vi "WriteTables1212(Host).vi"(1 "Select Channel":u16(ring) items=["CH 1", "CH 2"], 2 "WavefArray":u16[](array[numeric])=[8192, 8210, 8229, 8247, 8266, 8284, 8302, 8321, 8339, 8358, 8376, 8394, 8413, 8431, 8450, 8468, 8486, 8505, 8523, 8542, 8560, 8578, 8597, 8615, 8633, 8652, 8670, 8688, 8707, 8725, 8743, 8762, 8780, 8798, 8817, 8835, 8853, 8872, 8890, 8908, 8926, 8945, 8963, 8981, 8999, 9018, 9036, 9054, 9072, 9091, 9109, 9127, 9145, 9163, 9181, 9200, 9218, 9236, 9254, 9272, 9290, 9308, 9326, 9344, 9363, 9381, 9399, 9417, 9435, 9453, 9471, 9489, 9507, 9525, 9543, 9560, 9578, 9596, 9614, 9632, 9650, 9668, 9686, 9703, 9721, 9739, 9757, 9775, 9792, 9810, 9828, 9845, 9863, 9881, 9898, 9916, 9934, 9951, 9969, 9986, 10004, 10022, 10039, 10057, 10074, 10092, 10109, 10126, 10144, 10161, 10179, 10196, 10213, 10231, 10248, 10265, 10283, 10300, 10317, 10334, 10351, 10369, 10386, 10403, 10420, 10437, 10454, 10471, 10488, 10505, 10522, 10539, 10556, 10573, 10590, 10607, 10623, 10640, 10657, 10674, 10691, 10707, 10724, 10741, 10757, 10774, 10791, 10807, 10824, 10840, 10857, 10873, 10890, 10906, 10923, 10939, 10955, 10972, 10988, 11004, 11020, 11037, 11053, 11069, 11085, 11101, 11117, 11133, 11149, 11165, 11181, 11197, 11213, 11229, 11245, 11261, 11277, 11292, 11308, 11324, 11340, 11355, 11371, 11386, 11402, 11418, 11433, 11449, 11464, 11479, 11495, 11510, 11525, 11541, 11556, 11571, 11586, 11602, 11617, 11632, 11647, 11662, 11677, 11692, 11707, 11722, 11737, 11751, 11766, 11781, 11796, 11810, 11825, 11840, 11854, 11869, 11883, 11898, 11912, 11927, 11941, 11956, 11970, 11984, 11998, 12013, 12027, 12041, 12055, 12069, 12083, 12097, 12111, 12125, 12139, 12153, 12166, 12180, 12194, 12208, 12221, 12235, 12249, 12262, 12276, 12289, 12303, 12316, 12329, 12343, 12356, 12369, 12382, 12395, 12409, 12422, 12435, 12448, 12461, 12474, 12486, 12499, 12512, 12525, 12537, 12550, 12563, 12575, 12588, 12600, 12613, 12625, 12638, 12650, 12662, 12675, 12687, 12699, 12711, 12723, 12735, 12747, 12759, 12771, 12783, 12795, 12807, 12818, 12830, 12842, 12853, 12865, 12876, 12888, 12899, 12911, 12922, 12933, 12945, 12956, 12967, 12978, 12989, 13000, 13011, 13022, 13033, 13044, 13055, 13066, 13076, 13087, 13098, 13108, 13119, 13129, 13140, 13150, 13160, 13171, 13181, 13191, 13201, 13211, 13221, 13231, 13241, 13251, 13261, 13271, 13281, 13290, 13300, 13310, 13319, 13329, 13338, 13348, 13357, 13367, 13376, 13385, 13394, 13403, 13413, 13422, 13431, 13440, 13448, 13457, 13466, 13475, 13484, 13492, 13501, 13509, 13518, 13526, 13535, 13543, 13551, 13560, 13568, 13576, 13584, 13592, 13600, 13608, 13616, 13624, 13632, 13639, 13647, 13655, 13662, 13670, 13677, 13685, 13692, 13699, 13707, 13714, 13721, 13728, 13735, 13742, 13749, 13756, 13763, 13770, 13777, 13783, 13790, 13797, 13803, 13810, 13816, 13822, 13829, 13835, 13841, 13847, 13854, 13860, 13866, 13872, 13878, 13883, 13889, 13895, 13901, 13906, 13912, 13917, 13923, 13928, 13934, 13939, 13944, 13949, 13955, 13960, 13965, 13970, 13975, 13980, 13984, 13989, 13994, 13999, 14003, 14008, 14012, 14017, 14021, 14025, 14030, 14034, 14038, 14042, 14046, 14050, 14054, 14058, 14062, 14066, 14069, 14073, 14077, 14080, 14084, 14087, 14091, 14094, 14097, 14100, 14104, 14107, 14110, 14113, 14116, 14119, 14122, 14124, 14127, 14130, 14132, 14135, 14137, 14140, 14142, 14145, 14147, 14149, 14151, 14153, 14155, 14157, 14159, 14161, 14163, 14165, 14167, 14168, 14170, 14171, 14173, 14174, 14176, 14177, 14178, 14180, 14181, 14182, 14183, 14184, 14185, 14186, 14186, 14187, 14188, 14189, 14189, 14190, 14190, 14191, 14191, 14191, 14192, 14192, 14192, 14192, 14192, 14192, 14192, 14192, 14192, 14191, 14191, 14191, 14190, 14190, 14189, 14189, 14188, 14187, 14186, 14186, 14185, 14184, 14183, 14182, 14181, 14180, 14178, 14177, 14176, 14174, 14173, 14171, 14170, 14168, 14167, 14165, 14163, 14161, 14159, 14157, 14155, 14153, 14151, 14149, 14147, 14145, 14142, 14140, 14137, 14135, 14132, 14130, 14127, 14124, 14122, 14119, 14116, 14113, 14110, 14107, 14104, 14100, 14097, 14094, 14091, 14087, 14084, 14080, 14077, 14073, 14069, 14066, 14062, 14058, 14054, 14050, 14046, 14042, 14038, 14034, 14030, 14025, 14021, 14017, 14012, 14008, 14003, 13999, 13994, 13989, 13984, 13980, 13975, 13970, 13965, 13960, 13955, 13949, 13944, 13939, 13934, 13928, 13923, 13917, 13912, 13906, 13901, 13895, 13889, 13883, 13878, 13872, 13866, 13860, 13854, 13847, 13841, 13835, 13829, 13822, 13816, 13810, 13803, 13797, 13790, 13783, 13777, 13770, 13763, 13756, 13749, 13742, 13735, 13728, 13721, 13714, 13707, 13699, 13692, 13685, 13677, 13670, 13662, 13655, 13647, 13639, 13632, 13624, 13616, 13608, 13600, 13592, 13584, 13576, 13568, 13560, 13551, 13543, 13535, 13526, 13518, 13509, 13501, 13492, 13484, 13475, 13466, 13457, 13448, 13440, 13431, 13422, 13413, 13403, 13394, 13385, 13376, 13367, 13357, 13348, 13338, 13329, 13319, 13310, 13300, 13290, 13281, 13271, 13261, 13251, 13241, 13231, 13221, 13211, 13201, 13191, 13181, 13171, 13160, 13150, 13140, 13129, 13119, 13108, 13098, 13087, 13076, 13066, 13055, 13044, 13033, 13022, 13011, 13000, 12989, 12978, 12967, 12956, 12945, 12933, 12922, 12911, 12899, 12888, 12876, 12865, 12853, 12842, 12830, 12818, 12807, 12795, 12783, 12771, 12759, 12747, 12735, 12723, 12711, 12699, 12687, 12675, 12662, 12650, 12638, 12625, 12613, 12600, 12588, 12575, 12563, 12550, 12537, 12525, 12512, 12499, 12486, 12474, 12461, 12448, 12435, 12422, 12409, 12395, 12382, 12369, 12356, 12343, 12329, 12316, 12303, 12289, 12276, 12262, 12249, 12235, 12221, 12208, 12194, 12180, 12166, 12153, 12139, 12125, 12111, 12097, 12083, 12069, 12055, 12041, 12027, 12013, 11998, 11984, 11970, 11956, 11941, 11927, 11912, 11898, 11883, 11869, 11854, 11840, 11825, 11810, 11796, 11781, 11766, 11751, 11737, 11722, 11707, 11692, 11677, 11662, 11647, 11632, 11617, 11602, 11586, 11571, 11556, 11541, 11525, 11510, 11495, 11479, 11464, 11449, 11433, 11418, 11402, 11386, 11371, 11355, 11340, 11324, 11308, 11292, 11277, 11261, 11245, 11229, 11213, 11197, 11181, 11165, 11149, 11133, 11117, 11101, 11085, 11069, 11053, 11037, 11020, 11004, 10988, 10972, 10955, 10939, 10923, 10906, 10890, 10873, 10857, 10840, 10824, 10807, 10791, 10774, 10757, 10741, 10724, 10707, 10691, 10674, 10657, 10640, 10623, 10607, 10590, 10573, 10556, 10539, 10522, 10505, 10488, 10471, 10454, 10437, 10420, 10403, 10386, 10369, 10351, 10334, 10317, 10300, 10283, 10265, 10248, 10231, 10213, 10196, 10179, 10161, 10144, 10126, 10109, 10092, 10074, 10057, 10039, 10022, 10004, 9986, 9969, 9951, 9934, 9916, 9898, 9881, 9863, 9845, 9828, 9810, 9792, 9775, 9757, 9739, 9721, 9703, 9686, 9668, 9650, 9632, 9614, 9596, 9578, 9560, 9543, 9525, 9507, 9489, 9471, 9453, 9435, 9417, 9399, 9381, 9363, 9344, 9326, 9308, 9290, 9272, 9254, 9236, 9218, 9200, 9181, 9163, 9145, 9127, 9109, 9091, 9072, 9054, 9036, 9018, 8999, 8981, 8963, 8945, 8926, 8908, 8890, 8872, 8853, 8835, 8817, 8798, 8780, 8762, 8743, 8725, 8707, 8688, 8670, 8652, 8633, 8615, 8597, 8578, 8560, 8542, 8523, 8505, 8486, 8468, 8450, 8431, 8413, 8394, 8376, 8358, 8339, 8321, 8302, 8284, 8266, 8247, 8229, 8210, 8192, 8174, 8155, 8137, 8118, 8100, 8082, 8063, 8045, 8026, 8008, 7990, 7971, 7953, 7934, 7916, 7898, 7879, 7861, 7842, 7824, 7806, 7787, 7769, 7751, 7732, 7714, 7696, 7677, 7659, 7641, 7622, 7604, 7586, 7567, 7549, 7531, 7512, 7494, 7476, 7458, 7439, 7421, 7403, 7385, 7366, 7348, 7330, 7312, 7293, 7275, 7257, 7239, 7221, 7203, 7184, 7166, 7148, 7130, 7112, 7094, 7076, 7058, 7040, 7021, 7003, 6985, 6967, 6949, 6931, 6913, 6895, 6877, 6859, 6841, 6824, 6806, 6788, 6770, 6752, 6734, 6716, 6698, 6681, 6663, 6645, 6627, 6609, 6592, 6574, 6556, 6539, 6521, 6503, 6486, 6468, 6450, 6433, 6415, 6398, 6380, 6362, 6345, 6327, 6310, 6292, 6275, 6258, 6240, 6223, 6205, 6188, 6171, 6153, 6136, 6119, 6101, 6084, 6067, 6050, 6033, 6015, 5998, 5981, 5964, 5947, 5930, 5913, 5896, 5879, 5862, 5845, 5828, 5811, 5794, 5777, 5761, 5744, 5727, 5710, 5693, 5677, 5660, 5643, 5627, 5610, 5593, 5577, 5560, 5544, 5527, 5511, 5494, 5478, 5461, 5445, 5429, 5412, 5396, 5380, 5364, 5347, 5331, 5315, 5299, 5283, 5267, 5251, 5235, 5219, 5203, 5187, 5171, 5155, 5139, 5123, 5107, 5092, 5076, 5060, 5044, 5029, 5013, 4998, 4982, 4966, 4951, 4935, 4920, 4905, 4889, 4874, 4859, 4843, 4828, 4813, 4798, 4782, 4767, 4752, 4737, 4722, 4707, 4692, 4677, 4662, 4647, 4633, 4618, 4603, 4588, 4574, 4559, 4544, 4530, 4515, 4501, 4486, 4472, 4457, 4443, 4428, 4414, 4400, 4386, 4371, 4357, 4343, 4329, 4315, 4301, 4287, 4273, 4259, 4245, 4231, 4218, 4204, 4190, 4176, 4163, 4149, 4135, 4122, 4108, 4095, 4081, 4068, 4055, 4041, 4028, 4015, 4002, 3989, 3975, 3962, 3949, 3936, 3923, 3910, 3898, 3885, 3872, 3859, 3847, 3834, 3821, 3809, 3796, 3784, 3771, 3759, 3746, 3734, 3722, 3709, 3697, 3685, 3673, 3661, 3649, 3637, 3625, 3613, 3601, 3589, 3577, 3566, 3554, 3542, 3531, 3519, 3508, 3496, 3485, 3473, 3462, 3451, 3439, 3428, 3417, 3406, 3395, 3384, 3373, 3362, 3351, 3340, 3329, 3318, 3308, 3297, 3286, 3276, 3265, 3255, 3244, 3234, 3224, 3213, 3203, 3193, 3183, 3173, 3163, 3153, 3143, 3133, 3123, 3113, 3103, 3094, 3084, 3074, 3065, 3055, 3046, 3036, 3027, 3017, 3008, 2999, 2990, 2981, 2971, 2962, 2953, 2944, 2936, 2927, 2918, 2909, 2900, 2892, 2883, 2875, 2866, 2858, 2849, 2841, 2833, 2824, 2816, 2808, 2800, 2792, 2784, 2776, 2768, 2760, 2752, 2745, 2737, 2729, 2722, 2714, 2707, 2699, 2692, 2685, 2677, 2670, 2663, 2656, 2649, 2642, 2635, 2628, 2621, 2614, 2607, 2601, 2594, 2587, 2581, 2574, 2568, 2562, 2555, 2549, 2543, 2537, 2530, 2524, 2518, 2512, 2506, 2501, 2495, 2489, 2483, 2478, 2472, 2467, 2461, 2456, 2450, 2445, 2440, 2435, 2429, 2424, 2419, 2414, 2409, 2404, 2400, 2395, 2390, 2385, 2381, 2376, 2372, 2367, 2363, 2359, 2354, 2350, 2346, 2342, 2338, 2334, 2330, 2326, 2322, 2318, 2315, 2311, 2307, 2304, 2300, 2297, 2293, 2290, 2287, 2284, 2280, 2277, 2274, 2271, 2268, 2265, 2262, 2260, 2257, 2254, 2252, 2249, 2247, 2244, 2242, 2239, 2237, 2235, 2233, 2231, 2229, 2227, 2225, 2223, 2221, 2219, 2217, 2216, 2214, 2213, 2211, 2210, 2208, 2207, 2206, 2204, 2203, 2202, 2201, 2200, 2199, 2198, 2198, 2197, 2196, 2195, 2195, 2194, 2194, 2193, 2193, 2193, 2192, 2192, 2192, 2192, 2192, 2192, 2192, 2192, 2192, 2193, 2193, 2193, 2194, 2194, 2195, 2195, 2196, 2197, 2198, 2198, 2199, 2200, 2201, 2202, 2203, 2204, 2206, 2207, 2208, 2210, 2211, 2213, 2214, 2216, 2217, 2219, 2221, 2223, 2225, 2227, 2229, 2231, 2233, 2235, 2237, 2239, 2242, 2244, 2247, 2249, 2252, 2254, 2257, 2260, 2262, 2265, 2268, 2271, 2274, 2277, 2280, 2284, 2287, 2290, 2293, 2297, 2300, 2304, 2307, 2311, 2315, 2318, 2322, 2326, 2330, 2334, 2338, 2342, 2346, 2350, 2354, 2359, 2363, 2367, 2372, 2376, 2381, 2385, 2390, 2395, 2400, 2404, 2409, 2414, 2419, 2424, 2429, 2435, 2440, 2445, 2450, 2456, 2461, 2467, 2472, 2478, 2483, 2489, 2495, 2501, 2506, 2512, 2518, 2524, 2530, 2537, 2543, 2549, 2555, 2562, 2568, 2574, 2581, 2587, 2594, 2601, 2607, 2614, 2621, 2628, 2635, 2642, 2649, 2656, 2663, 2670, 2677, 2685, 2692, 2699, 2707, 2714, 2722, 2729, 2737, 2745, 2752, 2760, 2768, 2776, 2784, 2792, 2800, 2808, 2816, 2824, 2833, 2841, 2849, 2858, 2866, 2875, 2883, 2892, 2900, 2909, 2918, 2927, 2936, 2944, 2953, 2962, 2971, 2981, 2990, 2999, 3008, 3017, 3027, 3036, 3046, 3055, 3065, 3074, 3084, 3094, 3103, 3113, 3123, 3133, 3143, 3153, 3163, 3173, 3183, 3193, 3203, 3213, 3224, 3234, 3244, 3255, 3265, 3276, 3286, 3297, 3308, 3318, 3329, 3340, 3351, 3362, 3373, 3384, 3395, 3406, 3417, 3428, 3439, 3451, 3462, 3473, 3485, 3496, 3508, 3519, 3531, 3542, 3554, 3566, 3577, 3589, 3601, 3613, 3625, 3637, 3649, 3661, 3673, 3685, 3697, 3709, 3722, 3734, 3746, 3759, 3771, 3784, 3796, 3809, 3821, 3834, 3847, 3859, 3872, 3885, 3898, 3910, 3923, 3936, 3949, 3962, 3975, 3989, 4002, 4015, 4028, 4041, 4055, 4068, 4081, 4095, 4108, 4122, 4135, 4149, 4163, 4176, 4190, 4204, 4218, 4231, 4245, 4259, 4273, 4287, 4301, 4315, 4329, 4343, 4357, 4371, 4386, 4400, 4414, 4428, 4443, 4457, 4472, 4486, 4501, 4515, 4530, 4544, 4559, 4574, 4588, 4603, 4618, 4633, 4647, 4662, 4677, 4692, 4707, 4722, 4737, 4752, 4767, 4782, 4798, 4813, 4828, 4843, 4859, 4874, 4889, 4905, 4920, 4935, 4951, 4966, 4982, 4998, 5013, 5029, 5044, 5060, 5076, 5092, 5107, 5123, 5139, 5155, 5171, 5187, 5203, 5219, 5235, 5251, 5267, 5283, 5299, 5315, 5331, 5347, 5364, 5380, 5396, 5412, 5429, 5445, 5461, 5478, 5494, 5511, 5527, 5544, 5560, 5577, 5593, 5610, 5627, 5643, 5660, 5677, 5693, 5710, 5727, 5744, 5761, 5777, 5794, 5811, 5828, 5845, 5862, 5879, 5896, 5913, 5930, 5947, 5964, 5981, 5998, 6015, 6033, 6050, 6067, 6084, 6101, 6119, 6136, 6153, 6171, 6188, 6205, 6223, 6240, 6258, 6275, 6292, 6310, 6327, 6345, 6362, 6380, 6398, 6415, 6433, 6450, 6468, 6486, 6503, 6521, 6539, 6556, 6574, 6592, 6609, 6627, 6645, 6663, 6681, 6698, 6716, 6734, 6752, 6770, 6788, 6806, 6824, 6841, 6859, 6877, 6895, 6913, 6931, 6949, 6967, 6985, 7003, 7021, 7040, 7058, 7076, 7094, 7112, 7130, 7148, 7166, 7184, 7203, 7221, 7239, 7257, 7275, 7293, 7312, 7330, 7348, 7366, 7385, 7403, 7421, 7439, 7458, 7476, 7494, 7512, 7531, 7549, 7567, 7586, 7604, 7622, 7641, 7659, 7677, 7696, 7714, 7732, 7751, 7769, 7787, 7806, 7824, 7842, 7861, 7879, 7898, 7916, 7934, 7953, 7971, 7990, 8008, 8026, 8045, 8063, 8082, 8100, 8118, 8137, 8155, 8174], 3 "error in":errorcluster, 4 "resource name":T1="RIO0" caption="RIO Device") -> (0 "error out":errorcluster)   [LabVIEW 2018]
uses:
  <vilib>/userdefined/High Color/nirio_resource_hc.ctl
  <vilib>/Utility/error.llb/Error Cluster From Error Code.vi
  <vilib>/rvi/errors/niLvFpgaAdjustHostInterfaceError.vi
  <vilib>/FPGAPlugInAG/Dynamic/niLvFpga_Close_Dynamic.vi
  <vilib>/rvi/interface/nirviReadWriteControl/nirviReadWriteControl.xnode
  <vilib>/rvi/interface/nirviCloseFPGA/nirviCloseFPGA.xnode
  NiFpgaLv.dll
  <vilib>/rvi/interface/Simulation/niFpgaSimulationCallBeginRW.vi
panel:
  out "FPGA Interface Out":refnum<k20>
  in  "FPGA Interface In":refnum<k20>
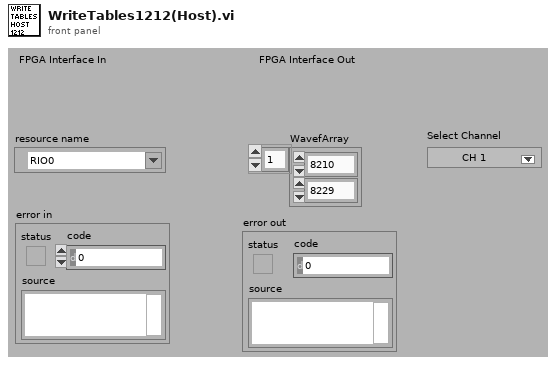
[diagram p1: front panel]
types:
  T1 = typedef "nirio_resource_hc.ctl" = tag
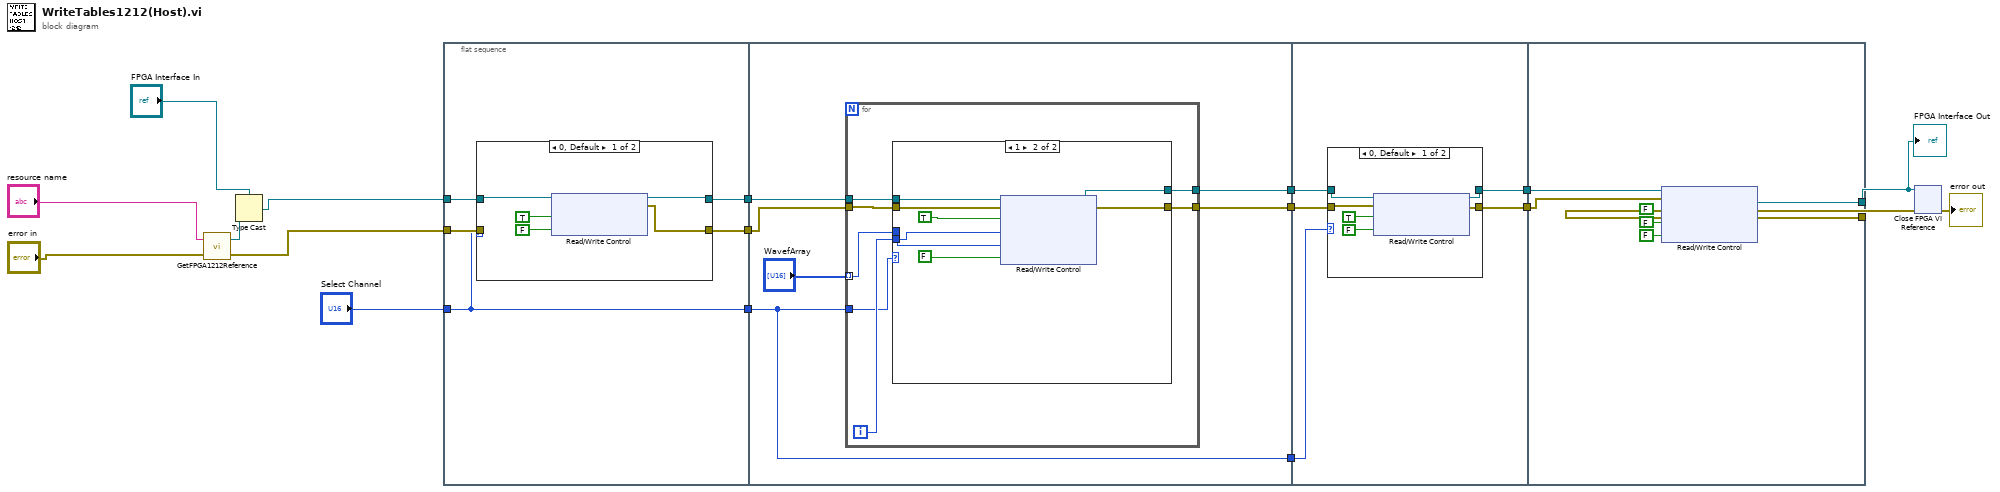
[diagram p0: block diagram]
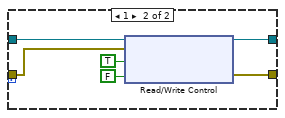
[diagram p2: hidden frame]
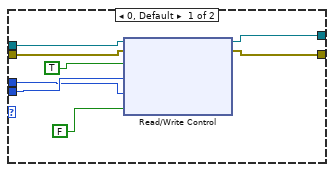
[diagram p3: hidden frame]
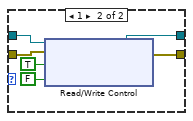
[diagram p4: hidden frame]
diagram:
  n1 = call "GetFPGA1212Reference.vi"("error in"="error in", "RIO Device IN"="resource name") -> ("error out"=w4:errorcluster, "FPGA VI Reference Out"=w1:refnum<k20>)
  n2 = Type Cast(type="FPGA Interface In", x=w1) -> (*(type *) &x=w3:refnum<k20>)
  n3 = flat-sequence {
    tunnel: w4 -> [w20]
    tunnel: w3 -> [w23]
    tunnel: [w22] -> w16
    tunnel: [w21] -> w15
    tunnel: "Select Channel" -> [w19]
    tunnel: [w19] -> w9
    tunnel: [w37] -> w14
    tunnel: [w36] -> w13
    tunnel: w16 -> [w40]
    tunnel: w15 -> [w39]
    tunnel: w9 -> [w35]
    tunnel: [w35] -> w8
    tunnel: w14 -> [w68]
    tunnel: [w66] -> w12
    tunnel: w13 -> [w67]
    tunnel: [w65] -> w11
    tunnel: w8 -> [w64]
    tunnel: [w87] -> w2
    tunnel: [w85] -> w17
    tunnel: w12 -> [w84]
    tunnel: w11 -> [w83]
    frame #0 {
      n4 = case shown="0, Default" w19 {
        tunnel: w23 -> [w28 w34]
        tunnel: [w27 w33] -> w22
        tunnel: [w26 w32] -> w21
        tunnel: w20 -> [_ w31]
        frame 0, Default {
          n5 = xnode "Read/Write Control"("FPGA VI Reference In"=w28, "WRITE MEM CH0"=TRUE ("WRITE MEM"), "SysReset"=FALSE) -> ("FPGA VI Reference Out"=w27:refnum<k20>, "error out"=w26:errorcluster)  [unwired: 1 in]
        }
        frame 1 {
          n6 = xnode "Read/Write Control"("FPGA VI Reference In"=w34, "error in"=w31, "WRITE MEM CH1"=TRUE ("WRITE MEM"), "SysReset"=FALSE) -> ("FPGA VI Reference Out"=w33:refnum<k20>, "error out"=w32:errorcluster)
        }
      }
    }
    frame #1 {
      n7 = for {
        tunnel: w39 -> [w46]
        tunnel: w40 -> [w47]
        tunnel: "WavefArray" -> [w45] mode=indexing
        tunnel: [w43] -> w37
        tunnel: [w42] -> w36
        tunnel: w35 -> [w41]
        i -> [w44]
        n8 = case shown="1" w41 {
          tunnel: w47 -> [w55 w63]
          tunnel: w46 -> [w54 w62]
          tunnel: w45 -> [w50 w61]
          tunnel: w44 -> [w51 w60]
          tunnel: [w53 w59] -> w43
          tunnel: [w52 w58] -> w42
          frame 0, Default {
            n9 = xnode "Read/Write Control"("FPGA VI Reference In"=w55, "error in"=w54, "WRITE MEM CH0"=TRUE ("WRITE MEM"), "WriteAddress"=w51, "WriteData"=w50, "SysReset"=FALSE) -> ("FPGA VI Reference Out"=w53:refnum<k20>, "error out"=w52:errorcluster)
          }
          frame 1 {
            n10 = xnode "Read/Write Control"("FPGA VI Reference In"=w63, "error in"=w62, "WRITE MEM CH1"=TRUE ("WRITE MEM"), "WriteAddress"=w60, "WriteData"=w61, "SysReset"=FALSE) -> ("FPGA VI Reference Out"=w59:refnum<k20>, "error out"=w58:errorcluster)
          }
        }
      }
    }
    frame #2 {
      n11 = case shown="0, Default" w64 {
        tunnel: w68 -> [w74 w80]
        tunnel: w67 -> [w71 w79]
        tunnel: [w73 w78] -> w66
        tunnel: [w72 w77] -> w65
        frame 0, Default {
          n12 = xnode "Read/Write Control"("FPGA VI Reference In"=w74, "error in"=w71, "WRITE MEM CH0"=TRUE ("WRITE MEM"), "SysReset"=FALSE) -> ("FPGA VI Reference Out"=w73:refnum<k20>, "error out"=w72:errorcluster)
        }
        frame 1 {
          n13 = xnode "Read/Write Control"("FPGA VI Reference In"=w80, "error in"=w79, "WRITE MEM CH1"=TRUE ("WRITE MEM"), "SysReset"=FALSE) -> ("FPGA VI Reference Out"=w78:refnum<k20>, "error out"=w77:errorcluster)
        }
      }
    }
    frame #3 {
      n14 = xnode "Read/Write Control"("FPGA VI Reference In"=w84, "error in"=w83, "WRITE MEM CH1"=FALSE ("WRITE MEM"), "SysReset"=FALSE, "WRITE MEM CH0"=FALSE ("WRITE MEM CH2")) -> ("FPGA VI Reference Out"=w87:refnum<k20>, "error out"=w85:errorcluster)
    }
  }
  n15 = xnode "Close FPGA VI Reference"("FPGA VI Reference In"=w2, "error in"=w17) -> ("error out"=→"error out":errorcluster)
  "FPGA Interface Out" <- w2
